vi "Move X-Y to L-.vi"(8 "error in (no error) 3":errorcluster) -> (0 "error out 3":errorcluster, 2 "cmd response":string, 3 "Enable response":string, 4 "Finished moving":bool)   [LabVIEW 2011]
panel:
  out "read_string 4":string
  out "read_string 3":string
  out "read_string 2":string
  out "read_string":string
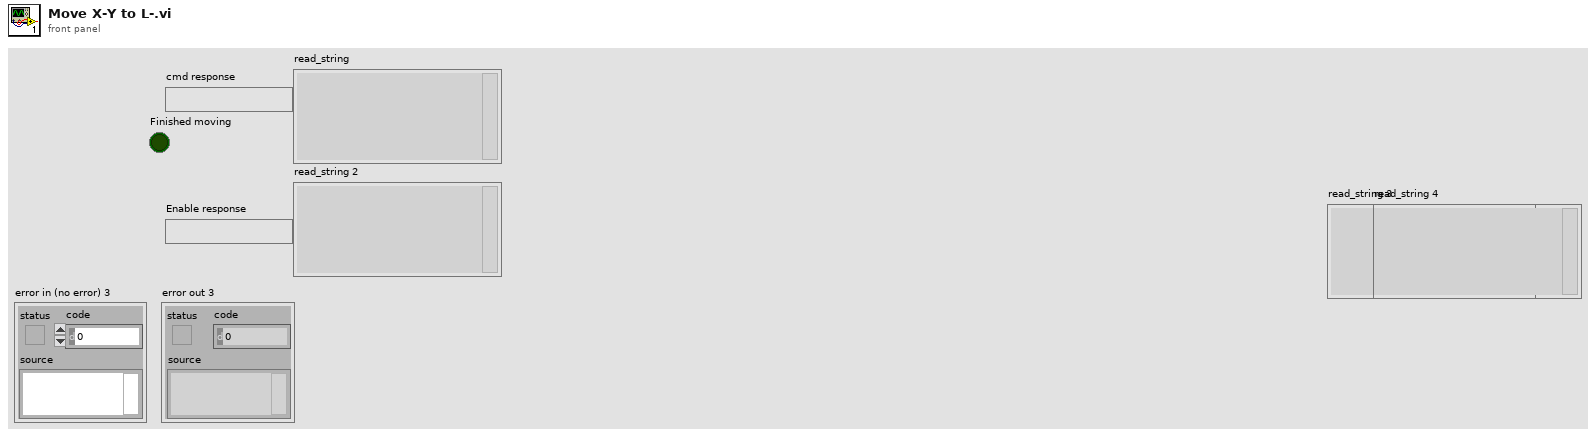
[diagram p1: front panel]
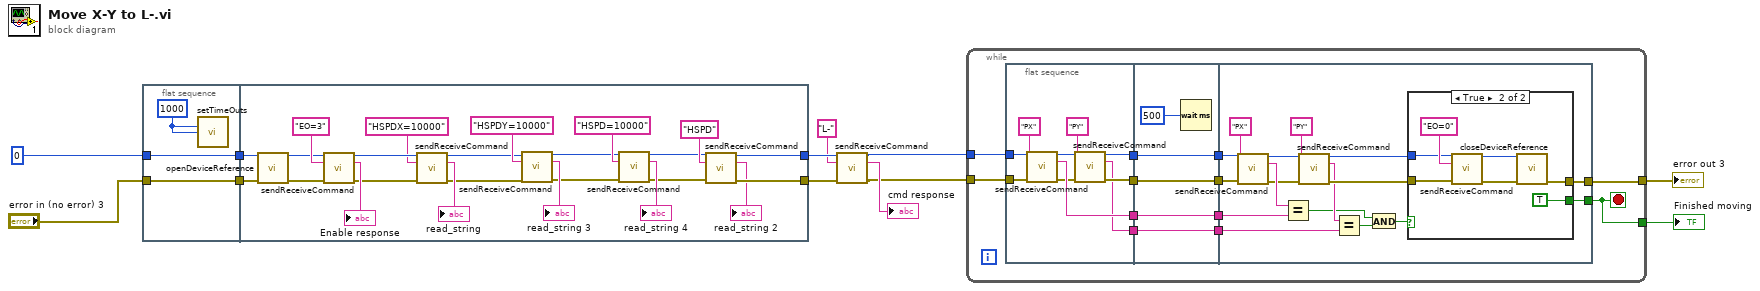
[diagram p0: block diagram]
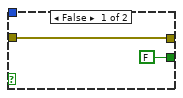
[diagram p2: hidden frame]
diagram:
  n1 = flat-sequence {
    tunnel: 0 -> [w14]
    tunnel: [w14] -> w9
    tunnel: "error in (no error) 3" -> [w13]
    tunnel: [w13] -> w8
    tunnel: w9 -> [w39]
    tunnel: w8 -> [w38]
    tunnel: [w33] -> w11
    tunnel: [w32] -> w7
    frame #0 {
      w15 = 1000 ("read_timeout")
      n2 = call "setTimeOuts.vi"("read_timeout (ms)"=w15, "write_timeout (ms)"=w15) -> ()  [unwired: 13 in, 1 out]
    }
    frame #1 {
      n3 = call "openDeviceReference.vi"("deviceIndex"=w39, "error in (no error)"=w38) -> ("reference"=w35:i32, "error out"=w34:errorcluster)  [unwired: 12 in]
      n4 = call "sendReceiveCommand.vi"("reference (in)"=w35, "write_string"="EO=3" ("raw_cmd 2"), "error in (no error)"=w34) -> ("reference (out)"=w31:i32, "read_string"=→"Enable response":string, "error out"=w30:errorcluster)  [unwired: 10 in]
      n5 = call "sendReceiveCommand.vi"("reference (in)"=w31, "write_string"="HSPDX=10000", "error in (no error)"=w30) -> ("reference (out)"=w23:i32, "read_string"=→"read_string":string, "error out"=w22:errorcluster)  [unwired: 10 in]
      n6 = call "sendReceiveCommand.vi"("reference (in)"=w23, "write_string"="HSPDY=10000", "error in (no error)"=w22) -> ("reference (out)"=w19:i32, "read_string"=→"read_string 3":string, "error out"=w18:errorcluster)  [unwired: 10 in]
      n7 = call "sendReceiveCommand.vi"("reference (in)"=w19, "write_string"="HSPD=10000", "error in (no error)"=w18) -> ("reference (out)"=w17:i32, "read_string"=→"read_string 4":string, "error out"=w16:errorcluster)  [unwired: 10 in]
      n8 = call "sendReceiveCommand.vi"("reference (in)"=w17, "write_string"="HSPD", "error in (no error)"=w16) -> ("reference (out)"=w33:i32, "read_string"=→"read_string 2":string, "error out"=w32:errorcluster)  [unwired: 10 in]
    }
  }
  n9 = call "sendReceiveCommand.vi"("reference (in)"=w11, "write_string"="L-", "error in (no error)"=w7) -> ("reference (out)"=w5:i32, "read_string"=→"cmd response":string, "error out"=w4:errorcluster)  [unwired: 10 in]
  n10 = while {
    tunnel: [w45] -> w6
    tunnel: w5 -> [w51]
    tunnel: w4 -> [w50]
    tunnel: [w40] -> w1
    stop <- w40 stop-if-true
    n11 = flat-sequence {
      tunnel: w51 -> [w60]
      tunnel: w50 -> [w59]
      tunnel: [w54] -> w49
      tunnel: [w53] -> w48
      tunnel: [w58] -> w43
      tunnel: [w52] -> w41
      tunnel: w49 -> [w66]
      tunnel: w48 -> [w65]
      tunnel: [w66] -> w47
      tunnel: [w65] -> w46
      tunnel: [w63] -> w44
      tunnel: w43 -> [w63]
      tunnel: [w62] -> w42
      tunnel: w41 -> [w62]
      tunnel: w47 -> [w82]
      tunnel: w46 -> [w81]
      tunnel: [w80] -> w45
      tunnel: [w79] -> w40
      tunnel: w44 -> [w77]
      tunnel: w42 -> [w69]
      frame #0 {
        n12 = call "sendReceiveCommand.vi"("reference (in)"=w60, "write_string"="PX" ("raw_cmd 2"), "error in (no error)"=w59) -> ("reference (out)"=w56:i32, "read_string"=w58:string, "error out"=w55:errorcluster)  [unwired: 10 in]
        n13 = call "sendReceiveCommand.vi"("reference (in)"=w56, "write_string"="PY" ("raw_cmd 2"), "error in (no error)"=w55) -> ("reference (out)"=w54:i32, "read_string"=w52:string, "error out"=w53:errorcluster)  [unwired: 10 in]
      }
      frame #1 {
        n14 = Wait (ms)(milliseconds to wait=500) -> ()  [unwired: 1 out]
      }
      frame #2 {
        n15 = call "sendReceiveCommand.vi"("reference (in)"=w82, "write_string"="PX" ("raw_cmd 2"), "error in (no error)"=w81) -> ("reference (out)"=w74:i32, "read_string"=w78:string, "error out"=w73:errorcluster)  [unwired: 10 in]
        n16 = Equal?(x=w78, y=w77) -> (x = y?=w67:bool)
        n17 = call "sendReceiveCommand.vi"("reference (in)"=w74, "write_string"="PY" ("raw_cmd 2"), "error in (no error)"=w73) -> ("reference (out)"=w72:i32, "read_string"=w68:string, "error out"=w71:errorcluster)  [unwired: 10 in]
        n18 = Equal?(x=w68, y=w69) -> (x = y?=w70:bool)
        n19 = And(x=w67, y=w70) -> (x .and. y?=w76:bool)
        n20 = case shown="True" w76 {
          tunnel: [w85 w92] -> w80
          tunnel: w71 -> [w85 w88]
          tunnel: w72 -> [_ w87]
          tunnel: [FALSE TRUE] -> w79
          frame False {
          }
          frame True {
            n21 = call "sendReceiveCommand.vi"("reference (in)"=w87, "write_string"="EO=0" ("raw_cmd 2"), "error in (no error)"=w88) -> ("reference (out)"=w90:i32, "error out"=w89:errorcluster)  [unwired: 10 in, 1 out]
            n22 = call "closeDeviceReference.vi"("reference"=w90, "error in (no error)"=w89) -> ("error out"=w92:errorcluster)  [unwired: 13 in]
          }
        }
      }
    }
  }
  "error out 3" <- w6
  "Finished moving" <- w1
